vi "Get Joystick Values.vi"(8 "error in (no error)":errorcluster, 11 "Demo Mode in":refnum<class "Demo Mode.lvclass">) -> (0 "error out":errorcluster, 2 "Joystick Data":T1, 3 "Demo Mode out":refnum<class "Demo Mode.lvclass">)   [LabVIEW 2019, in "Joysticks.lvlib" / "Demo Mode.lvclass"]
doc: "Use this method to get the joystick values in a cluster you can use for your application.\n\nModify the Type Def that this VI resturns to fit the controls needed for the robot.\n\nThis class is specificly for demos, where dunctionality is limited for 2 main controlers for saftey and ease of use, an a 3rd controler can overide and perform more advanced functions"
uses:
  Demo Mode.lvclass
  C:/Users/Public/Documents/Infinite Recharge/src robot/Classes/Joysticks/Joysticks.lvclass
  Controls/JoystickData.ctl
  Demo Mode.lvclass/Demo Mode.ctl
  Joysticks.lvclass/Joysticks.ctl
  Public Methods/Read Sensitivity(x).vi
  Public Methods/Read Sensitivity(y).vi
  <vilib>/Rock Robotics/WPI/Utilities/WPI_GetSetVariantRefNum.vi
  Private Methods/POV Conditioning.vi
  Joysticks.lvclass
  Two Drivers/Two Drivers.lvclass
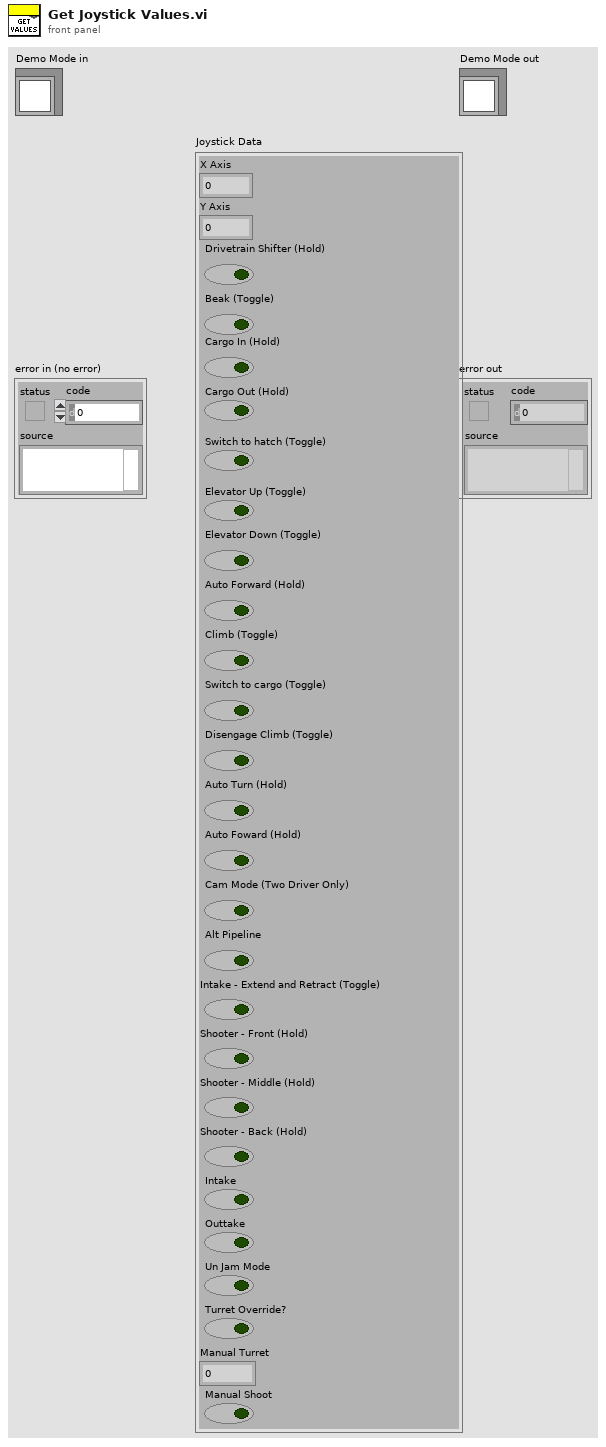
[diagram p1: front panel]
types:
  T1 = typedef "Joysticks.lvlib/Joysticks.lvclass/JoystickData.ctl" = cluster{"X Axis ":dbl, "Y Axis":dbl, "Drivetrain Shifter (Hold)":bool, "Beak (Toggle)":bool, "Cargo In (Hold)":bool, "Cargo Out (Hold)":bool, "Switch to hatch (Toggle)":bool, "Elevator Up (Toggle)":bool, "Elevator Down (Toggle)":bool, "Auto Forward (Hold)":bool, "Climb (Toggle)":bool, "Switch to cargo (Toggle)":bool, "Disengage Climb (Toggle)":bool, "Auto Turn (Hold)":bool, "Auto Foward (Hold)":bool, "Cam Mode (Two Driver Only)":bool, "Alt Pipeline":bool, "Intake - Extend and Retract (Toggle)":bool, "Shooter - Front (Hold)":bool, "Shooter - Middle (Hold)":bool, "Shooter - Back (Hold)":bool, "Intake":bool, "Outtake":bool, "Un Jam Mode":bool, "Turret Override?":bool, "Manual Turret":dbl, "Manual Shoot":bool}
  T2 = typedef "WPI_JoystickDevRef.ctl" = cluster{"Device":T3}
  T3 = typedef "WPI_JoystickDeviceEnum.ctl" = enum16{"USB 0", "USB 1", "USB 2", "USB 3", "USB 4", "USB 5"}
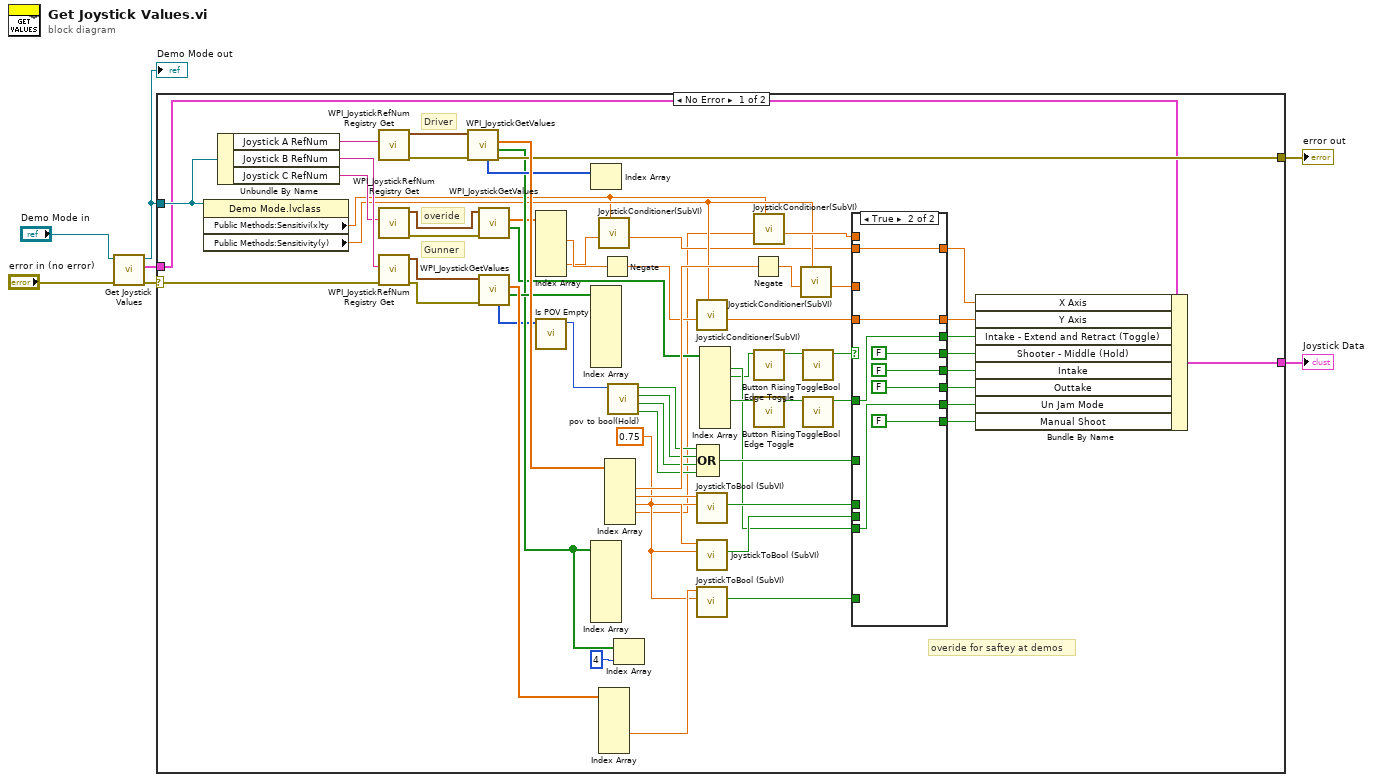
[diagram p0: block diagram]
diagram:
  n1 = call-parent "Get Joystick Values.vi"("error in (no error)"="error in (no error)", "Joysticks in"="Demo Mode in") -> ("error out"=w6:errorcluster, "Joystick Data"=w7:T1, "Joysticks out"=w3:refnum<class "Demo Mode.lvclass">)  [unwired: 7 in]
  "Demo Mode out" <- w3
  n2 = case shown="No Error" w6 {
    selector: w6 -> [w63 w87]
    tunnel: [w58 w87] -> w2
    tunnel: w3 -> [w55 _]
    tunnel: [w67 _] -> w1
    tunnel: w7 -> [w54 _]
    frame No Error {
      w45 = 0.75 ("y")
      # "overide for saftey at demos"
      # "overide"
      # "Gunner"
      # "Driver"
      n3 = property class="Demo Mode.lvclass"(reference=w55) -> ("Public Methods:Sensitivi(x)ty"=w13:dbl, "Public Methods:Sensitivity(y)"=w14:dbl)  [unwired: 1 in, 2 out]
      n4 = Unbundle By Name(w55) -> ("Joystick A RefNum"=w69:string, "Joystick B RefNum"=w61:string, "Joystick C RefNum"=w40:string)
      n5 = call <vilib>:"WPI_JoystickRefNum Registry Get.vi"("refnum name"=w69) -> ("error out"=w70:errorcluster, "JoystickDevRef"=w68:T2)  [unwired: 9 in]
      n6 = call <vilib>:"WPI_JoystickRefNum Registry Get.vi"("refnum name"=w40) -> ("error out"=w43:errorcluster, "JoystickDevRef"=w44:T2)  [unwired: 9 in]
      n7 = call <vilib>:"WPI_JoystickRefNum Registry Get.vi"("error in (no error)"=w63, "refnum name"=w61) -> ("error out"=w62:errorcluster, "JoystickDevRef"=w64:T2)  [unwired: 8 in]
      n8 = call <vilib>:"WPI_JoystickGetValues.vi"("error in (no error)"=w70, "JoystickDevRef"=w68) -> ("error out"=w58:errorcluster, "Buttons"=w53:bool[], "Axes"=w66:dbl[], "POVs"=w57:i16[])  [unwired: 5 in, 1 out]
      n9 = call <vilib>:"WPI_JoystickGetValues.vi"("error in (no error)"=w43, "JoystickDevRef"=w44) -> ("Buttons"=w41:bool[], "Axes"=w42:dbl[])  [unwired: 5 in, 3 out]
      n10 = call <vilib>:"WPI_JoystickGetValues.vi"("error in (no error)"=w62, "JoystickDevRef"=w64) -> ("Buttons"=w59:bool[], "Axes"=w60:dbl[], "POVs"=w49:i16[])  [unwired: 5 in, 2 out]
      n11 = Index Array(array=w42) -> (element #2=w15:dbl, element #5=w12:dbl)  [unwired: 6 in, 4 out]
      n12 = call "Is POV Empty.vi"("POVs"=w49) -> ("Numeric"=w48:i16)  [unwired: 10 in]
      n13 = Index Array(array=w57) -> ()  [unwired: 1 in, 1 out]
      n14 = Index Array(array=w59) -> ()  [unwired: 8 in, 8 out]
      n15 = Index Array(array=w53) -> ()  [unwired: 8 in, 8 out]
      n16 = call "JoystickConditioner(SubVI).vi"("Sensitivity"=w13, "joystick axis"=w12) -> ("output"=w11:dbl)  [unwired: 9 in]
      n17 = Index Array(array=w60) -> (element #4=w46:dbl)  [unwired: 6 in, 5 out]
      n18 = Negate(x=w15) -> (-x=w16:dbl)
      n19 = Index Array(array=w66) -> (element #2=w65:dbl, element #3=w50:dbl, element #4=w51:dbl, element #5=w8:dbl)  [unwired: 6 in, 2 out]
      n20 = call "pov to bool(Hold).vi"("Numeric"=w48) -> ("Left"=w35:bool, "Down"=w36:bool, "Up"=w37:bool, "Right"=w38:bool)  [unwired: 7 in]
      n21 = Index Array(array=w53, index=4) -> ()  [unwired: 1 out]
      n22 = call "JoystickConditioner(SubVI).vi"("Sensitivity"=w14, "joystick axis"=w16) -> ("output"=w10:dbl)  [unwired: 9 in]
      n23 = Compound Arithmetic op=OR(w38, w37, w36, w35) -> (w31:bool)
      n24 = call "JoystickToBool (SubVI).vi"("Threshold"=w45, "Axis"=w50) -> ("Joy Forward"=w30:bool)  [unwired: 8 in, 1 out]
      n25 = call "JoystickToBool (SubVI).vi"("Threshold"=w45, "Axis"=w51) -> ("Joy Forward"=w29:bool)  [unwired: 8 in, 1 out]
      n26 = call "JoystickToBool (SubVI).vi"("Threshold"=w45, "Axis"=w46) -> ("Joy Forward"=w27:bool)  [unwired: 8 in, 1 out]
      n27 = Index Array(array=w41) -> (element #1=w28:bool, element #2=w18:bool, element #5=w39:bool)  [unwired: 8 in, 5 out]
      n28 = Negate(x=w65) -> (-x=w56:dbl)
      n29 = call "JoystickConditioner(SubVI).vi"("Sensitivity"=w13, "joystick axis"=w8) -> ("output"=w34:dbl)  [unwired: 9 in]
      n30 = call "Button Rising Edge Toggle.vi"("Button"=w18) -> ("Rising edge?"=w19:bool)  [unwired: 10 in]
      n31 = call "Button Rising Edge Toggle.vi"("Button"=w39) -> ("Rising edge?"=w47:bool)  [unwired: 10 in]
      n32 = call "JoystickConditioner(SubVI).vi"("Sensitivity"=w14, "joystick axis"=w56) -> ("output"=w33:dbl)  [unwired: 9 in]
      n33 = call "ToggleBool.vi"("Boolean"=w19) -> ("toggled bool"=w17:bool)  [unwired: 10 in]
      n34 = call "ToggleBool.vi"("Boolean"=w47) -> ("toggled bool"=w32:bool)  [unwired: 10 in]
      n35 = case shown="True" w17 {
        tunnel: w34 -> [w78 _]
        tunnel: w33 -> [w77 _]
        tunnel: w32 -> [w76 w86]
        tunnel: w31 -> [w75 _]
        tunnel: w30 -> [w74 _]
        tunnel: w29 -> [w73 _]
        tunnel: w28 -> [w72 w85]
        tunnel: w27 -> [w71 _]
        tunnel: [w78 w80] -> w9
        tunnel: [w77 w79] -> w26
        tunnel: [w76 w86] -> w25
        tunnel: [w75 FALSE] -> w24
        tunnel: [w74 FALSE] -> w23
        tunnel: [w73 FALSE] -> w22
        tunnel: [w72 w85] -> w21
        tunnel: [w71 FALSE] -> w20
        tunnel: w11 -> [_ w80]
        tunnel: w10 -> [_ w79]
        frame False {
        }
        frame True {
        }
      }
      n36 = Bundle By Name(cluster=w54, "X Axis"=w9, "Y Axis"=w26, "Intake - Extend and Retract (Toggle)"=w25, "Shooter - Middle (Hold)"=w24, "Intake"=w23, "Outtake"=w22, "Un Jam Mode"=w21, "Manual Shoot"=w20) -> (w67:T1)
    }
    frame Error {
    }
  }
  "error out" <- w2
  "Joystick Data" <- w1
